vi "czujka_temperatury.vi"(5 "id pin":T1(ring), 6 "connection in":refnum<k31>) -> (0 "sending error":errorcluster, 1 "check buffer error":errorcluster, 2 "temperature":dbl, 3 "connection out":refnum<k31>, 4 "reapons char error":errorcluster)   [LabVIEW 2012]
uses:
  meas_date.vi
panel:
  out "check buffer error 2":errorcluster
  out "command id":u8
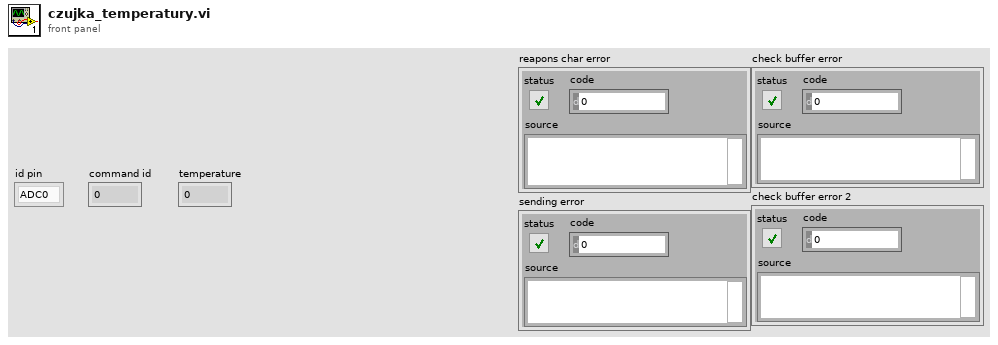
[diagram p1: front panel]
types:
  T1 = enum16{"ADC0", "ADC1", "ADC2", "ADC3", "ADC4", "ADC5", "ADC6", "ADC7"}
  T2 = cluster{"param":u64, "count":i32, "name":string}[]
  T3 = cluster{"id":u8, "name":string, "params":cluster{"name":string, "count":u8}[], "respons char":string[]}[]
  T4 = cluster{"received values[0]":u8, "received values[1]":u8, "received values[2]":u8, "received values[3]":u8, "received values[4]":u8, "received values[5]":u8, "received values[6]":u8, "received values[7]":u8, "received values[8]":u8}
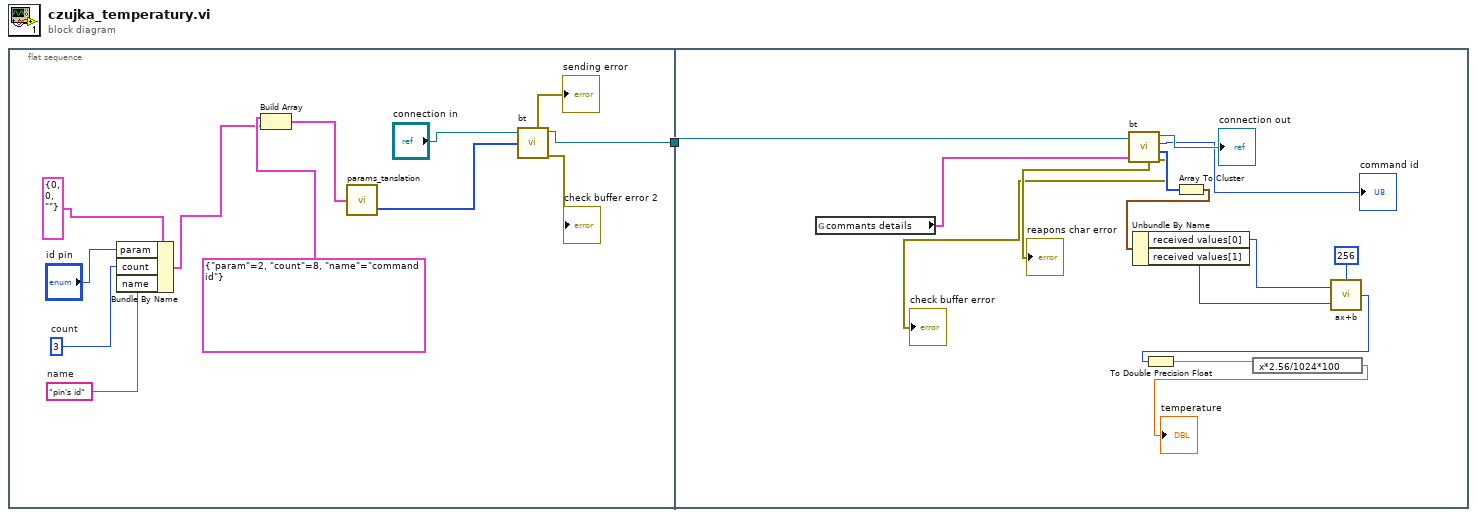
[diagram p0: block diagram]
diagram:
  n1 = flat-sequence {
    tunnel: [w7] -> w1
    tunnel: w1 -> [w27]
    frame #0 {
      w10 = u8 3  # count
      w11 = "pin's id"  # name
      n2 = Bundle By Name(cluster=cluster{"param":u64, "count":u8, "name":string} {"param"=0, "count"=0, "name"=""} ("Cluster"), "param"="id pin", "count"=w10, "name"=w11) -> (w5:cluster{"param":u64, "count":u8, "name":string})
      n3 = Build Array(cluster{"param":i32, "count":i32, "name":string} {"param"=2, "count"=8, "name"="command id"} ("Cluster"), w5) -> (w4:T2)
      n4 = call "params_tanslation.vi"("params"=w4) -> ("tablica charow (u8)"=w8:u8[])  [unwired: 1 out]
      n5 = call "bt.vi"("sending command"=w8, "connection in"="connection in") -> ("check buffer error"=→"check buffer error 2":errorcluster, "sending error"=→"sending error":errorcluster, "connection out"=w7:refnum<k31>)  [unwired: 1 in, 3 out]
    }
    frame #1 {
      n6 = global read "meas_date.vi" "commants details"() -> (w19:T3)
      n7 = call "bt.vi"("commants details"=w19, "connection in"=w27) -> ("check buffer error"=→"check buffer error":errorcluster, "reapons char error"=→"reapons char error":errorcluster, "received values"=w21:u8[], "income command id"=→"command id":u8, "connection out"=→"connection out":refnum<k31>)  [unwired: 1 in, 1 out]
      n8 = Array To Cluster(array=w21) -> (cluster=w22:T4)
      n9 = Unbundle By Name(w22) -> ("received values[0]"=w15:u8, "received values[1]"=w14:u8)
      n10 = call "ax+b.vi"("x"=256, "b"=w14, "a"=w15) -> ("y"=w24:i32)
      n11 = To Double Precision Float(number=w24) -> (double precision float=w25:dbl)
      n12 = expression code="x*2.56/1024*100"(w25) -> (→"temperature":dbl)
    }
  }
